vi "test Parse File Info_2.vi"(11 "Test Case In":refnum<class "test EDS.lvclass">) -> (0 "error out":errorcluster, 3 "Test Case Out":refnum<class "test EDS.lvclass">)   [LabVIEW 2024, in "test EDS.lvclass"]
uses:
  test EDS.lvclass
  C:/Program Files/National Instruments/LabVIEW 2024/vi.lib/Astemes/LUnit/Test Case.lvclass
  Core/EDS/EDS.lvclass
  <vilib>/PNR/JSONtext Object Serialization/Generic Object Serializer/Generic Object Serializer.lvclass
  C:/Program Files/National Instruments/LabVIEW 2024/vi.lib/JDP Science/JSONtext/LVClass Serializer/JSONtext LVClass Serializer.lvclass
  <vilib>/PNR/JSONtext Object Serialization/Generic Object Serializer/Type Name Handling.ctl
  <vilib>/PNR/JSONtext Object Serialization/Generic Object Serializer/Generic Object Serializer.lvclass/Generic Object Serializer.ctl
  Core/EDS/EDS.lvclass/EDS.ctl
  <vilib>/Astemes/LUnit/Test Case.lvclass/Test Case.ctl
  99df47cb-525e-4171-a825-741cf93afc66.vi
  4993e8ee-a06a-463a-9684-69129f64d5ce.vi
  <vilib>/PNR/JSONtext Object Serialization/Generic Object Serializer/Write Type Name Handling.vi
  <vilib>/Astemes/LUnit/Append Pass Result.vi
  <vilib>/Astemes/LUnit/Append Fail Result.vi
  <vilib>/Astemes/LUnit/Describe Comparison.vi
  4993e8ee-a06a-463a-9684-69129f64d5ce.vi/9c5d11cd-9439-4240-a1ee-d9baace9c924.vi
  <vilib>/Astemes/LUnit/Run In UI.vi
  <vilib>/Utility/error.llb/Clear Errors.vi
  <vilib>/JDP Science/JSONtext/Variant to JSON Text.vi
  <vilib>/Astemes/LUnit/Describe Variant.vi
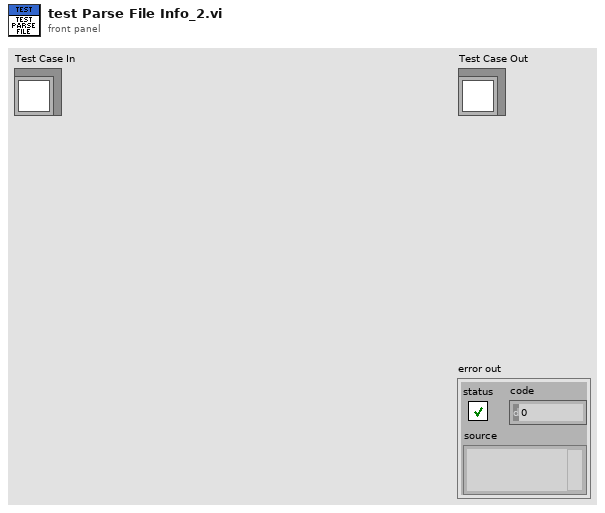
[diagram p1: front panel]
types:
  T1 = typedef "Generic Object Serializer.lvclass/Type Name Handling.ctl" = enum16{"None", "Inline"}
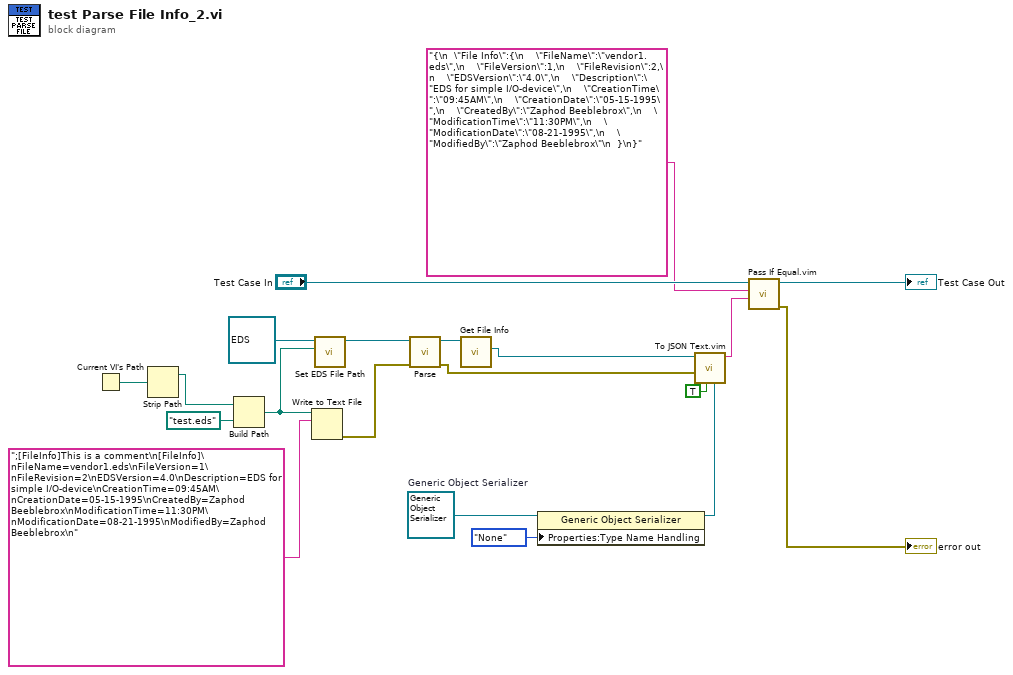
[diagram p0: block diagram]
diagram:
  w7 = refnum<class "Generic Object Serializer.lvclass"> refnum  # Generic Object Serializer
  n1 = Current VI's Path() -> (path=w15:path)
  n2 = Strip Path(path=w15) -> (stripped path=w14:path)  [unwired: 1 out]
  n3 = Build Path(base path=w14, name or relative path=path "test.eds") -> (appended path=w13:path)
  n4 = Write to Text File(file (use dialog)=w13, text=";[FileInfo]This is a comment\n[FileInfo]\nFileName=vendor1.eds\nFileVersion=1\nFileRevision=2\nEDSVersion=4.0\nDescription=EDS for simple I/O-device\nCreationTime=09:45AM\nCreationDate=05-15-1995\nCreatedBy=Zaphod Beeblebrox\nModificationTime=11:30PM\nModificationDate=08-21-1995\nModifiedBy=Zaphod Beeblebrox\n") -> (error out=w11:errorcluster)  [unwired: 2 in, 2 out]
  n5 = call "Set EDS File Path.vi"("EDS File Path"=w13, "EDS in"=refnum<class "EDS.lvclass"> refnum ("EDS.lvlib:EDS.lvclass")) -> ("EDS out"=w16:refnum<class "EDS.lvclass">)  [unwired: 9 in]
  n6 = call "Parse.vi"("error in"=w11, "EDS in"=w16) -> ("error out"=w4:errorcluster, "EDS out"=w9:refnum<class "EDS.lvclass">)  [unwired: 8 in]
  n7 = call "Get File Info.vi"("EDS in"=w9) -> ("File Info"=w3:refnum<class "File Info.lvclass">)  [unwired: 9 in, 1 out]
  n8 = property class="Generic Object Serializer"(reference=w7, "Properties:Type Name Handling"=Type_Name_Handling."None" ("Type Name Handling")) -> (reference out=w6:refnum<class "Generic Object Serializer.lvclass">)  [unwired: 1 in, 1 out]
  n9 = call "To JSON Text.vim"("LVClass Serializer"=w6, "Pretty Print?"=TRUE, "error in (no error)"=w4, "Anything"=w3) -> ("<JSON>"=w2:string)  [unwired: 6 in, 1 out]
  n10 = call "Pass If Equal.vim"("Actual"=w2, "Expected"="{\n  \"File Info\":{\n    \"FileName\":\"vendor1.eds\",\n    \"FileVersion\":1,\n    \"FileRevision\":2,\n    \"EDSVersion\":\"4.0\",\n    \"Description\":\"EDS for simple I/O-device\",\n    \"CreationTime\":\"09:45AM\",\n    \"CreationDate\":\"05-15-1995\",\n    \"CreatedBy\":\"Zaphod Beeblebrox\",\n    \"ModificationTime\":\"11:30PM\",\n    \"ModificationDate\":\"08-21-1995\",\n    \"ModifiedBy\":\"Zaphod Beeblebrox\"\n  }\n}" ("<JSON>"), "LUnit Test Case In"="Test Case In") -> ("error out"=→"error out":errorcluster, "LUnit Test Case Out"=→"Test Case Out":refnum<class "test EDS.lvclass">)  [unwired: 7 in]
